vi "QueuedMessageHandler.vi"() -> ()   [LabVIEW 2020]
panel:
  out "error out":errorcluster
  in  "error in":errorcluster
  in  "stop":bool
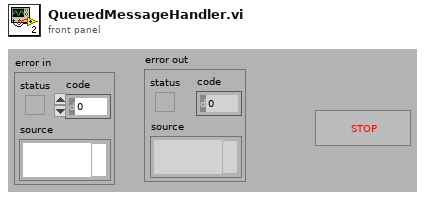
[diagram p1: front panel]
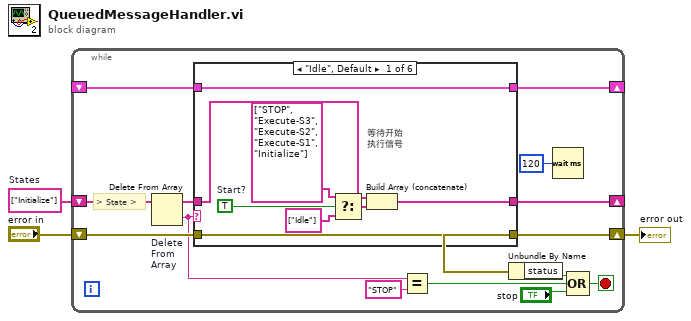
[diagram p0: block diagram]
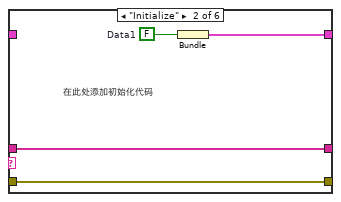
[diagram p2: hidden frame]
diagram:
  w1 = string[] ["Initialize"]  # States
  n1 = while {
    shift-right: [w17] -> _
    shift-left: w1 -> [w9]
    shift-right: [w11] -> w2
    shift-left: "error in" -> [w12]
    shift-right: [w5] -> _
    shift-left: _ -> [w4]
    stop <- w14 stop-if-true
    # "> State >"
    n2 = Delete From Array "Delete\nFrom\nArray"(array=w9) -> (deleted portion=w8:string, array with subset deleted=w7:string[])  [unwired: 2 in]
    n3 = case shown="\"Idle\", Default" w8 {
      tunnel: [w22 w28 w32 w35 w37 w40] -> w17
      tunnel: w12 -> [w25 w29 w31 w34 w38 w41]
      tunnel: [w25 w29 w31 w34 w38 w41] -> w11
      tunnel: w7 -> [w19 w28 w32 w35 w37 w40]
      tunnel: [w18 w26 w30 w33 w36 w39] -> w5
      tunnel: w4 -> [w18 _ w30 w33 w36 w39]
      frame "Idle", Default {
        w24 = TRUE  # Start?
        # "等待开始\n执行信号"
        n4 = Select(t=string[] ["STOP", "Execute-S3", "Execute-S2", "Execute-S1", "Initialize"] ("States"), s=w24, f=string[] ["Idle"] ("States")) -> (s? t:f=w23:string[])
        n5 = Build Array (concatenate) "Build Array"(w19, w23) -> (w22:string[])
      }
      frame "Initialize" {
        w27 = FALSE  # Data1
        # "在此处添加初始化代码"
        n6 = Bundle("Data1"=w27) -> (w26:cluster{"Data1":bool})  [unwired: 1 in]
      }
      frame "Execute-S1" {
        # "在此处添加测试S1阶段的代码"
      }
      frame "Execute-2" {
        # "在此处添加测试S2阶段的代码"
      }
      frame "Execute-3" {
        # "在此处添加测试S3阶段的代码"
      }
      frame "STOP" {
        # "在此处添加现场清理代码"
      }
    }
    n7 = Equal?(x=w8, y="STOP") -> (x = y?=w13:bool)
    n8 = Unbundle By Name(w11) -> ("status"=w10:bool)
    n9 = Wait (ms)(milliseconds to wait=u32 120) -> ()  [unwired: 1 out]
    n10 = Compound Arithmetic op=OR(w10, w13, "stop") -> (w14:bool)
  }
  "error out" <- w2
